vi "test.ingest_dataflash.vi"   [LabVIEW 2020]
uses:
  datasources/dataset/dataset.lvclass
  datasources/dataset/dataset.lvclass/dataset.ctl
  Nominal Client/Nominal Client.lvclass/Nominal Client.ctl
  nominal types/workspace/workspace.lvclass/workspace.ctl
  81c5314d-0c17-4e40-9591-806fc92e59be.vi
  40e2c779-94f0-4ff6-913c-6196809b7e71.vi
  datasources/dataset/datasetName.set.vi
  Nominal Client/private_data.set.vi
  nominal types/workspace/id.get.vi
  nominal types/workspace/rid.get.vi
  <vilib>/AdvancedString/1D String Array to Delimited String.vi
  Nominal Client/workspace.set.vi
  datasources/gcs/gcs.lvclass
  C:/code/labview-client/lv_src/datasources/source/source.lvclass
  datasources/s3/s3.lvclass
  datasources/source/create_s3.vi
  datasources/source/create_gcs.vi
  <vilib>/Utility/file.llb/Application Directory.vi
  <vilib>/Utility/error.llb/Error Cluster From Error Code.vi
  Nominal Client/Palette Items/who_am_i.vi
  datasources/target/create_new.vi
  datasources/target/create_from_existing.vi
  Nominal Client/ingest_dataflash.vi
  Nominal Client/workspace_cache.get_from_rid.vi
  Nominal Client/workspace_cache.get.vi
  User/User.lvclass
  Nominal Client/Nominal Client.lvclass
  nominal types/workspace/workspace.lvclass
  submodules/reqwest-labview/lv-src/reqwest/reqwest.lvclass
  datasources/source/source.lvclass
  nominal types/channelConfig/channelConfig.lvclass
  datasources/target/target.lvclass
  nominal types/properties/properties.lvclass
  C:/code/labview-client/lv_src/datasources/payload/payload.lvclass
  C:/code/labview-client/lv_src/datasources/s3/s3.lvclass
  C:/code/labview-client/lv_src/datasources/gcs/gcs.lvclass
types:
  T1 = cluster{"dataset":refnum<class "dataset.lvclass">, "channelConfig":refnum<class "channelConfig.lvclass">}
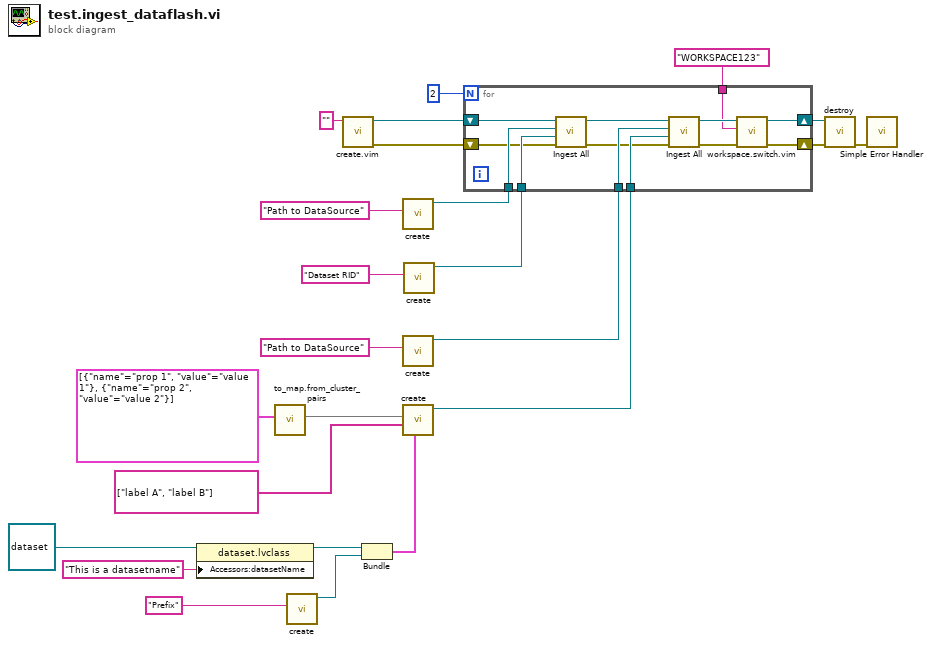
[diagram p0: block diagram]
diagram:
  n1 = property class="dataset.lvclass"(reference=refnum<class "dataset.lvclass"> refnum ("dataset"), "Accessors:datasetName"="This is a datasetname" ("datasetName")) -> (reference out=w15:refnum<class "dataset.lvclass">)  [unwired: 1 in, 1 out]
  n2 = call "to_map.from_cluster_pairs.vi"("properties (cluster pairs)"=cluster{"name":string, "value":string}[] [{"name"="prop 1", "value"="value 1"}, {"name"="prop 2", "value"="value 2"}] ("properties")) -> ("properties (map)"=w1:map{string, string})  [unwired: 10 in]
  n3 = call "create.vi"("prefixTreeDelimiter"="Prefix") -> ("channelConfig"=w9:refnum<class "channelConfig.lvclass">)  [unwired: 10 in]
  n4 = call "create.vim"("API Token (string or path)"="") -> ("error out"=w19:errorcluster, "Nominal Client"=w20:refnum<class "Nominal Client.lvclass">)  [unwired: 8 in, 1 out]
  n5 = Bundle("dataset"=w15, "channelConfig"=w9) -> (w6:T1)  [unwired: 1 in]
  n6 = call-poly "create.vi"("Path"="Path to DataSource") -> ("source"=w13:refnum<class "s3.lvclass">)  [unwired: 10 in]
  n7 = call-poly "create.vi"("Path"="Path to DataSource") -> ("source"=w11:refnum<class "gcs.lvclass">)  [unwired: 10 in]
  n8 = call-poly "create.vi"("Optional"=w6, "Labels"=string[] ["label A", "label B"] ("labels"), "Properties"=w1) -> ("New Target"=w5:refnum<class "target.lvclass">)  [unwired: 8 in]
  n9 = call-poly "create.vi"("dataset RID"="Dataset RID" ("RID")) -> ("Existing Target"=w7:refnum<class "target.lvclass">)  [unwired: 10 in]
  n10 = for {
    N: 2 -> [_]
    tunnel: w7 -> [w37]
    tunnel: w13 -> [w36]
    tunnel: w11 -> [w35]
    tunnel: w5 -> [w34]
    shift-right: [w27] -> w22
    shift-left: w19 -> [w31]
    shift-right: [w26] -> w24
    shift-left: w20 -> [w30]
    tunnel: "WORKSPACE123" ("RID") -> [w25]
    n11 = call-poly "Ingest All.vi"("error in"=w31, "Target"=w37, "Source"=w36, "Nominal Client in"=w30) -> ("error out"=w32:errorcluster, "Nominal Client out"=w33:refnum<class "Nominal Client.lvclass">)  [unwired: 4 in, 2 out]
    n12 = call-poly "Ingest All.vi"("error in"=w32, "Target"=w34, "Source"=w35, "Nominal Client in"=w33) -> ("error out"=w28:errorcluster, "Nominal Client out"=w29:refnum<class "Nominal Client.lvclass">)  [unwired: 4 in, 2 out]
    n13 = call "workspace.switch.vim"("error in"=w28, "Workspace (Object, RID, Path)"=w25, "Nominal Client in"=w29) -> ("error out"=w27:errorcluster, "Nominal Client out"=w26:refnum<class "Nominal Client.lvclass">)  [unwired: 7 in]
  }
  n14 = call "destroy.vi"("error in"=w22, "Nominal Client"=w24) -> ("error out"=w4:errorcluster)  [unwired: 9 in]
  n15 = call <vilib>:"Simple Error Handler.vi"("error in (no error)"=w4) -> ()  [unwired: 4 in, 5 out]
